vi "initializeStyleCollection.vi"(8 "error in (no error)":errorcluster, 11 "MS-Excel in":refnum<class "MS-Excel.lvclass">) -> (0 "error out":errorcluster, 3 "MS-Excel out":refnum<class "MS-Excel.lvclass">)   [LabVIEW 2020, in "LabVIEW NPOI.lvlib" / "MS-Excel.lvclass"]
uses:
  MS-Excel.lvclass
  MS-Excel.lvclass/MS-Excel.ctl
  Document/Document.lvclass
  D:/Benjamin/Documents/Perso/Code/WC/LabVIEW_NPOI/lib/NPOI 2.1.1/NPOI.dll
  lib/NPOI 2.1.1/NPOI.dll
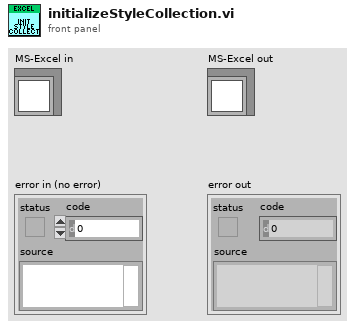
[diagram p1: front panel]
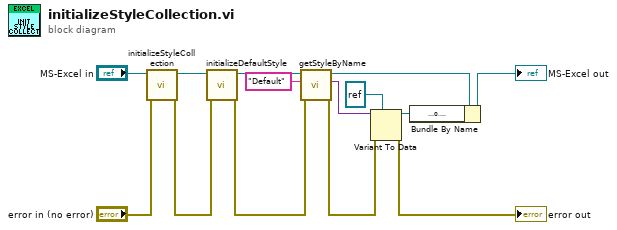
[diagram p0: block diagram]
diagram:
  n1 = call-parent "initializeStyleCollection.vi"("error in (no error)"="error in (no error)", "Document in"="MS-Excel in") -> ("error out"=w10:errorcluster, "Document out"=w12:refnum<class "MS-Excel.lvclass">)  [unwired: 8 in]
  n2 = call "initializeDefaultStyle.vi"("error in (no error)"=w10, "MS-Excel in"=w12) -> ("error out"=w8:errorcluster, "MS-Excel out"=w11:refnum<class "MS-Excel.lvclass">)  [unwired: 8 in]
  n3 = call-dynamic "getStyleByName.vi"("error in (no error)"=w8, "Style Name"="Default", "MS-Excel in"=w11) -> ("error out"=w2:errorcluster, "Style"=w5:variant, "MS-Excel out"=w9:refnum<class "MS-Excel.lvclass">)  [unwired: 6 in]
  n4 = Variant To Data(error in=w2, type=refnum<k24> refnum ("Cell Style"), Variant=w5) -> (data=w3:refnum<k24>, error out=→"error out":errorcluster)
  n5 = Bundle By Name(cluster=w9, "Cell Style"=w3) -> (→"MS-Excel out":refnum<class "MS-Excel.lvclass">)
